vi "stat_f_s3.vi"(5 "Array of Waveform":waveform(dbl)[](array[waveform])) -> (1 "Array 2":waveform(i16)[][](array[waveform]), 2 "sync":waveform(i16))   [LabVIEW 2010]
uses:
  <vilib>/Waveform/WDTOps.llb/WDT Get Waveform Subset DBL (LV80).vi
panel:
  out "final stops":i32[](array[numeric])
  out "final starts":i32[](array[numeric])
  out "sorted stops":i32[](array[numeric])
  out "sorted starts":i32[](array[numeric])
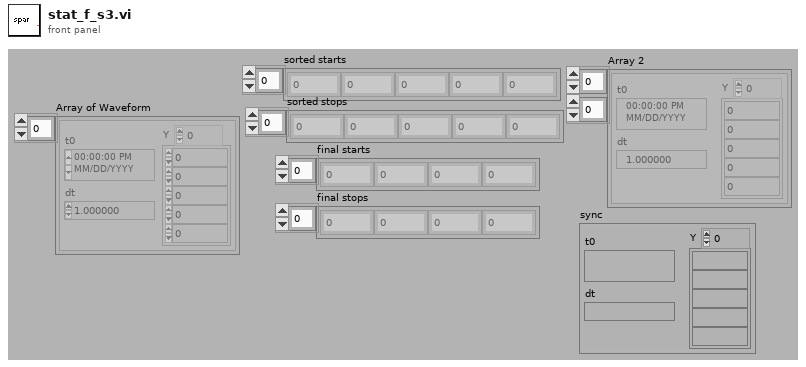
[diagram p1: front panel]
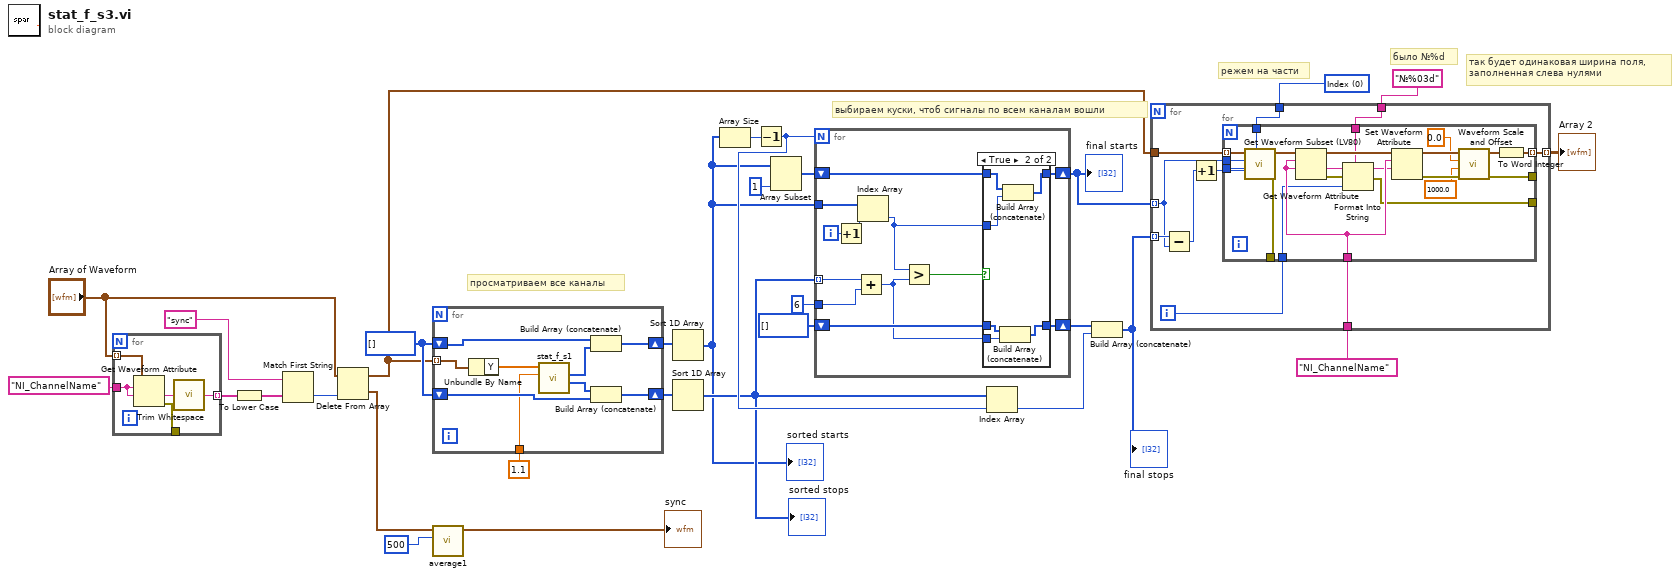
[diagram p0: block diagram]
diagram:
  w28 = u16 0 items=["Index", "Relative Time"] ("Mode")
  w14 = i32[] []
  # "так будет одинаковая ширина поля, \nзаполненная слева нулями"
  # "было №%d"
  # "режем на части"
  # "выбираем куски, чтоб сигналы по всем каналам вошли"
  # "просматриваем все каналы"
  n1 = for {
    tunnel: "Array of Waveform" -> [w35] mode=indexing
    tunnel: "NI_ChannelName" ("name") -> [w33]
    tunnel: [w32] -> w10 mode=indexing
    tunnel: [w31] -> _
    n2 = Get Waveform Attribute(5:w33, 6:w33, 7:w35) -> (0:w31:errorcluster, 1:w34:string)  [unwired: 1 in, 2 out]
    n3 = call <vilib>:"Trim Whitespace.vi"("string"=w34) -> ("trimmed string"=w32:string)  [unwired: 1 in]
  }
  n4 = To Lower Case(string=w10) -> (all lower case string=w5:string[])
  n5 = Match First String(2:w5, 3:"sync" ("name")) -> (0:w8:i32)  [unwired: 1 out]
  n6 = Delete From Array(array="Array of Waveform", index=w8) -> (deleted portion=w2:waveform(dbl), array with subset deleted=w6:waveform(dbl)[])  [unwired: 1 in]
  n7 = for {
    tunnel: w6 -> [w43] mode=indexing
    shift-right: [w41] -> w13
    shift-left: w14 -> [w40]
    shift-right: [w38] -> w15
    shift-left: w14 -> [w37]
    tunnel: 1.1 ("kD") -> [w36]
    n8 = Unbundle By Name(w43) -> ("Y"=w44:dbl[])
    n9 = call "stat_f_s1.vi"("kD"=w36, "Y"=w44) -> ("stops"=w39:i32[], "starts"=w42:i32[])  [unwired: 3 in, 1 out]
    n10 = Build Array (concatenate)(w40, w42) -> (w41:i32[])
    n11 = Build Array (concatenate)(w39, w37) -> (w38:i32[])
  }
  n12 = call "average1.vi"("Size"=u32 500, "Signal"=w2) -> ("Mean"=→"sync":waveform(i16))  [unwired: 5 in]
  n13 = Sort 1D Array(array=w13) -> (sorted array=w18:i32[])
  "sorted starts" <- w18
  n14 = Sort 1D Array(array=w15) -> (sorted array=w22:i32[])
  "sorted stops" <- w22
  n15 = Array Size(array=w18) -> (size(s)=w19:i32)
  n16 = Decrement(x=w19) -> (x-1=w23:i32)
  n17 = Array Subset(array=w18, length=1) -> (w16:i32[])  [unwired: 1 in]
  n18 = for {
    N: w23 -> [_]
    tunnel: w18 -> [w56]
    tunnel: w22 -> [w49] mode=indexing
    shift-right: [w53] -> w26
    shift-left: w16 -> [w52]
    tunnel: 6 ("length") -> [w50]
    shift-right: [w48] -> w25
    shift-left: i32[] [] -> [w47]
    i -> [w54]
    n19 = Increment(x=w54) -> (x+1=w55:i32)
    n20 = Add(x=w49, y=w50) -> (x+y=w46:i32)
    n21 = Index Array(array=w56, index=w55) -> (element=w45:i32)
    n22 = Greater?(x=w45, y=w46) -> (0:w51:bool)
    n23 = case shown="True" w51 {
      tunnel: w45 -> [_ w64]
      tunnel: [w58 w63] -> w53
      tunnel: w52 -> [w58 w62]
      tunnel: w46 -> [_ w61]
      tunnel: [w57 w60] -> w48
      tunnel: w47 -> [w57 w59]
      frame False {
      }
      frame True {
        n24 = Build Array (concatenate)(w59, w61) -> (w60:i32[])
        n25 = Build Array (concatenate)(w62, w64) -> (w63:i32[])
      }
    }
  }
  "final starts" <- w26
  n26 = Index Array(array=w22, index=w23) -> (element=w24:i32)
  n27 = Build Array (concatenate)(w25, w24) -> (w27:i32[])
  "final stops" <- w27
  n28 = for {
    tunnel: w26 -> [w72] mode=indexing
    tunnel: w27 -> [w74] mode=indexing
    tunnel: w6 -> [w73]
    tunnel: [w70] -> w30 mode=indexing
    tunnel: w28 -> [w68]
    tunnel: "NI_ChannelName" ("name") -> [w67]
    tunnel: "№%03d" ("format string") -> [w65]
    i -> [w66]
    n29 = Subtract(x=w74, y=w72) -> (x-y=w71:i32)
    n30 = Increment(x=w71) -> (x+1=w69:i32)
    n31 = for {
      tunnel: w73 -> [w95] mode=indexing
      tunnel: [w81] -> w70 mode=indexing
      tunnel: w72 -> [w94]
      tunnel: w69 -> [w93]
      tunnel: w68 -> [w92]
      tunnel: w67 -> [w89]
      tunnel: w66 -> [w88]
      tunnel: w65 -> [w85]
      tunnel: [w83] -> _
      tunnel: [w82] -> _
      tunnel: [w77] -> _
      n32 = call-poly <vilib>:"Get Waveform Subset (LV80).vi"("start/duration format"=w92, "duration"=w93, "start samples/time"=w94, "waveform in"=w95) -> ("error out"=w83:errorcluster, "waveform out"=w91:waveform(dbl))  [unwired: 2 in, 2 out]
      n33 = Get Waveform Attribute(5:w89, 6:w89, 7:w91) -> (0:w84:errorcluster, 1:w87:string, 3:w90:waveform(dbl))  [unwired: 1 in, 1 out]
      n34 = Format Into String(format string=w85, initial string=w87, error in=w84, w88) -> (resulting string=w86:string, error out=w82:errorcluster)
      n35 = Set Waveform Attribute(5:w86, 6:w89, 7:w90) -> (0:w80:errorcluster, 3:w79:waveform(dbl))  [unwired: 1 in, 1 out]
      n36 = call <vilib>:"Waveform Scale and Offset.vi"("error in (no error)"=w80, "scale"=1000.0, "offset"=0.0, "waveform in"=w79) -> ("error out"=w77:errorcluster, "waveform out"=w78:waveform(dbl))  [unwired: 6 in]
      n37 = To Word Integer(number=w78) -> (16bit integer=w81:waveform(i16))
    }
  }
  "Array 2" <- w30
